vi "Create DISCONNECT Packet.vi"(5 "DISCONNECT in":refnum<class "DISCONNECT.lvclass">, 8 "error in (no error)":errorcluster) -> (0 "error out":errorcluster, 2 "Bytes Stream":u8[](array[numeric]) format="%08b", 3 "DISCONNECT":refnum<class "DISCONNECT.lvclass">)   [LabVIEW 2013, in "MQTT_Control_Packets.lvlib" / "DISCONNECT.lvclass"]
uses:
  DISCONNECT.lvclass
  ControlPacket/ControlPacket.lvclass/ControlPacket.ctl
  ControlPacket/ControlPacket.lvclass
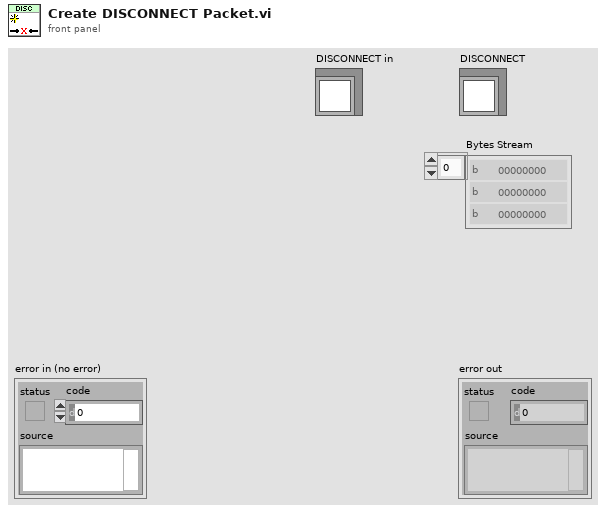
[diagram p1: front panel]
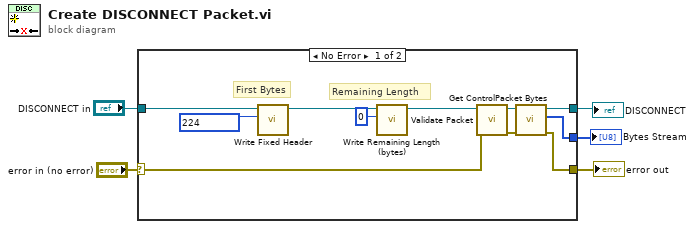
[diagram p0: block diagram]
diagram:
  n1 = case shown="No Error" "error in (no error)" {
    selector: "error in (no error)" -> [w11 w18]
    tunnel: [w7 w18] -> w2
    tunnel: [w9 w17] -> w3
    tunnel: "DISCONNECT in" -> [w16 w17]
    tunnel: [w6 _] -> w1
    frame No Error {
      # "Remaining Length"
      # "First Bytes"
      n2 = call "Write Fixed Header.vi"("Fixed Header"=u8 224, "ControlPacket in"=w16) -> ("ControlPacket out"=w15:refnum<class "DISCONNECT.lvclass">)  [unwired: 9 in]
      n3 = call "Write Remaining Length (bytes).vi"("Remaining Length (bytes)"=u32 0, "ControlPacket in"=w15) -> ("ControlPacket out"=w12:refnum<class "DISCONNECT.lvclass">)  [unwired: 9 in]
      n4 = call "Validate Packet.vi"("error in (no error)"=w11, "ControlPacket in"=w12) -> ("error out"=w8:errorcluster, "ControlPacket out"=w10:refnum<class "DISCONNECT.lvclass">)  [unwired: 8 in]
      n5 = call "Get ControlPacket Bytes.vi"("error in (no error)"=w8, "ControlPacket"=w10) -> ("error out"=w7:errorcluster, "Bytes Stream"=w6:u8[], "ControlPacket dup"=w9:refnum<class "DISCONNECT.lvclass">)  [unwired: 6 in, 1 out]
    }
    frame Error {
    }
  }
  "error out" <- w2
  "DISCONNECT" <- w3
  "Bytes Stream" <- w1
